vi "Read Current open project.vi"(11 "BuildManager in":refnum<class "BuildManager.lvclass">) -> (2 "Current open project":refnum<vi>, 3 "BuildManager out":refnum<class "BuildManager.lvclass">)   [LabVIEW 2019, in "SolutionBuilder.lvlib" / "BuildManager.lvclass"]
uses:
  BuildManager.lvclass
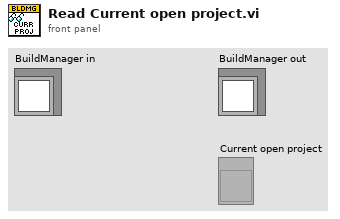
[diagram p1: front panel]
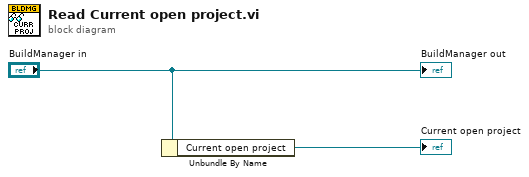
[diagram p0: block diagram]
diagram:
  n1 = Unbundle By Name("BuildManager in") -> ("Current open project"=→"Current open project":refnum<vi>)
  "BuildManager out" <- "BuildManager in"
